vi "ErrorMessage.vi"(11 "ErrorCode":i32) -> (3 "Message":string)   [LabVIEW 2018]
uses:
  <vilib>/Utility/file.llb/Read Delimited Spreadsheet (string).vi
panel:
  # "<機能>\nErrorCodeからエラーメッセージを取得する。\nメッセージはErrorCode.csvに定義する。"
  # "Input"
  # "Output"
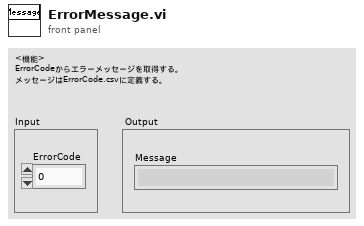
[diagram p1: front panel]
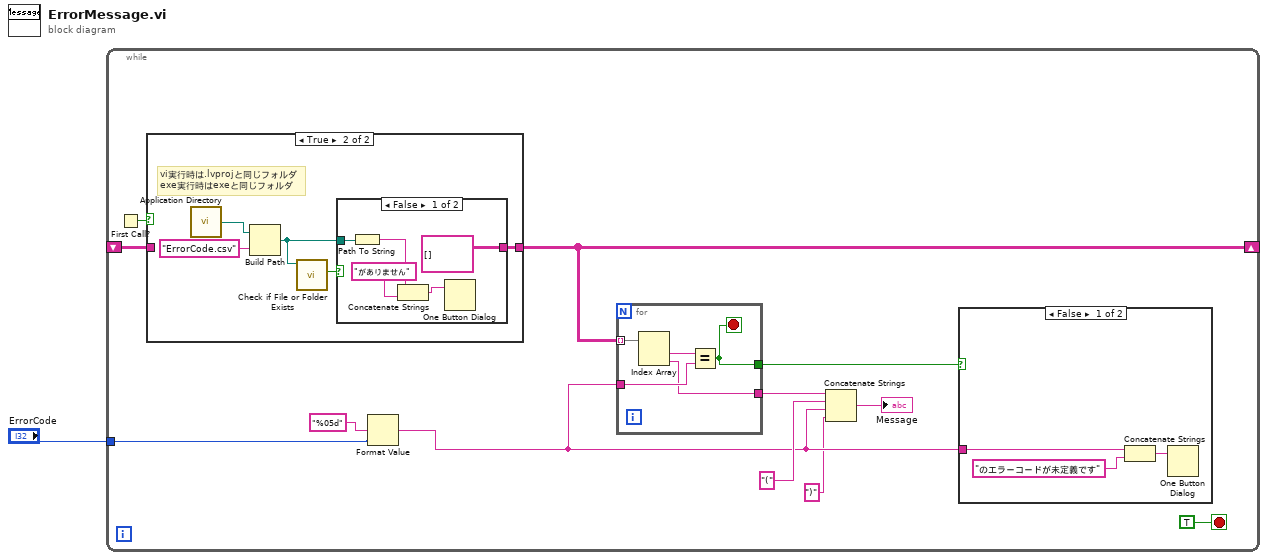
[diagram p0: block diagram]
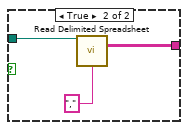
[diagram p3: hidden frame]
diagram:
  n1 = while {
    shift-right: [w10] -> _
    shift-left: _ -> [w11]
    tunnel: "ErrorCode" -> [w7]
    stop <- TRUE stop-if-true
    n2 = First Call?() -> (First Call?: T/F=w9:bool)
    n3 = case shown="TRUE" w9 {
      tunnel: [w14 w19] -> w10
      tunnel: w11 -> [w14 _]
      frame False {
      }
      frame True {
        # "vi実行時は.lvprojと同じフォルダ\nexe実行時はexeと同じフォルダ"
        n4 = call <vilib>:"Application Directory.vi"() -> ("Application Directory"=w15:path)
        n5 = Build Path(base path=w15, name or relative path="ErrorCode.csv" ("名前または相対パス")) -> (appended path=w17:path)
        n6 = call <vilib>:"Check if File or Folder Exists.vi"("path"=w17) -> ("file or folder exists?"=w16:bool)  [unwired: 8 in, 2 out]
        n7 = case shown="FALSE" w16 {
          tunnel: [string[][] [] ("all rows") w26] -> w19
          tunnel: w17 -> [w23 w25]
          frame False {
            n8 = Path To String(path=w23) -> (string=w22:string)
            n9 = Concatenate Strings(w22, "がありません" ("文字列")) -> (w21:string)
            n10 = One Button Dialog(message=w21) -> ()  [unwired: 1 in, 1 out]
          }
          frame True {
            n11 = call-poly <vilib>:"Read Delimited Spreadsheet.vi"("file path (dialog if empty)"=w25, "delimiter (\\t)"="," ("delimiter (\\t)")) -> ("all rows"=w26:string[][])  [unwired: 8 in, 5 out]
          }
        }
      }
    }
    n12 = Format Value(format string="%05d" ("形式文字列"), value (0)=w7) -> (output string=w4:string)  [unwired: 1 in]
    n13 = for {
      tunnel: w10 -> [w35] mode=indexing
      tunnel: w4 -> [w33]
      tunnel: [w31] -> w12
      tunnel: [w32] -> w6
      stop <- w31 stop-if-true
      n14 = Index Array(array=w35) -> (element #1=w34:string, element #2=w32:string)  [unwired: 2 in]
      n15 = Equal?(x=w34, y=w33) -> (x = y?=w31:bool)
    }
    n16 = Concatenate Strings(w6, "(" ("文字列"), w4, ")" ("文字列")) -> (→"Message":string)
    n17 = case shown="FALSE" w12 {
      tunnel: w4 -> [w30 _]
      frame False {
        n18 = Concatenate Strings(w30, "のエラーコードが未定義です" ("文字列")) -> (w28:string)
        n19 = One Button Dialog(message=w28) -> ()  [unwired: 1 in, 1 out]
      }
      frame True {
      }
    }
  }
